vi "Test3He.vi"() -> ()   [LabVIEW 2018]
panel:
  in  "stop":bool
  out "error out":errorcluster
  out "3HePressure (Torr)":string
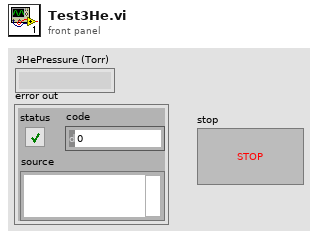
[diagram p1: front panel]
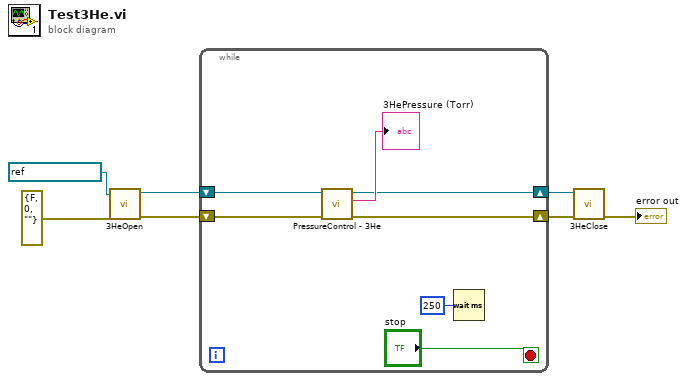
[diagram p0: block diagram]
diagram:
  n1 = call "3HeOpen.vi"("error in (no error)"=errorcluster {"status"=FALSE, "code"=0, "source"=""}, "VISA resource name"=refnum<visa-resource-name> "3HePressure") -> ("error out"=w6:errorcluster, "VISA resource name out"=w7:refnum<visa-resource-name>)  [unwired: 8 in]
  n2 = while {
    shift-right: [w12] -> w4
    shift-left: w7 -> [w13]
    shift-right: [w10] -> w5
    shift-left: w6 -> [w11]
    stop <- "stop" stop-if-true
    n3 = call "PressureControl - 3He.vi"("error in (no error)"=w11, "VISA resource name"=w13) -> ("error out"=w10:errorcluster, "3HePressure (Torr)"=→"3HePressure (Torr)":string, "VISA resource name out"=w12:refnum<visa-resource-name>)  [unwired: 7 in]
    n4 = Wait (ms)(milliseconds to wait=u32 250) -> ()  [unwired: 1 out]
  }
  n5 = call "3HeClose.vi"("error in (no error)"=w5, "VISA resource name"=w4) -> ("error out"=→"error out":errorcluster)  [unwired: 9 in]
